vi "Resolution effect on SFDR.vi"() -> ()   [LabVIEW 2019]
uses:
  <vilib>/Analysis/4window.llb/windowTd.ctl
  <vilib>/measure/maspectr.llb/Power Spectrum and PSD Export Mode.ctl
  <vilib>/measure/maspectr.llb/FFT Power Spectrum and PSD for N Chan.vi
  <vilib>/measure/NI_MABase.lvlib
  <vilib>/measure/NI_MAPro.lvlib
  <vilib>/Analysis/NI_AALPro.lvlib
panel:
  out "Power spectrum":cluster{"f0":dbl, "df":dbl, "magnitude":dbl[]}[](graph)
  in  "sampling info":cluster{"Fs":dbl, "#s":dbl}={"Fs"=3072000000.0, "#s"=16000.0}
  in  "amplitude":dbl=0.5 format="%0.2p"
  in  "Fc":dbl=500000000.0 format="%#_6pHz"
  out "noise level":dbl=-81.98970004336019 format="%#_gdbm"
  in  "BW":dbl=2000000000.0 format="%#_6pHz"
  in  "Noise density":dbl=-155.0 format="%#_gdbm/Hz"
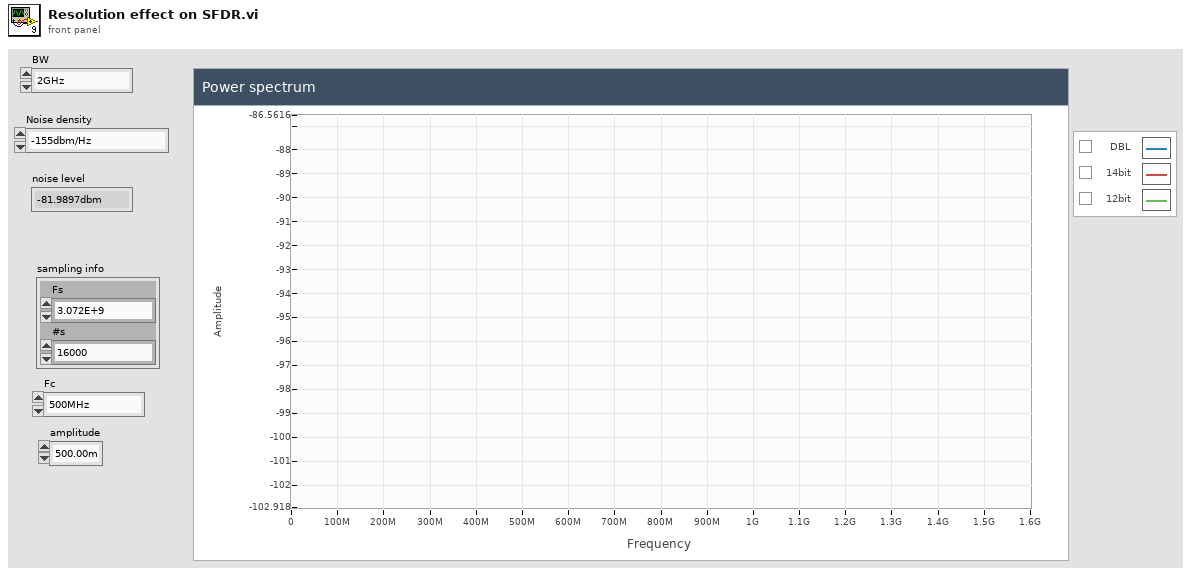
[diagram p1: front panel]
types:
  T1 = typedef "NI_MAPro.lvlib/Power Spectrum and PSD Export Mode.ctl" = u16
  T2 = typedef "NI_AALPro.lvlib/windowTd.ctl" = u32
  T3 = enum16{"Sine Wave", "Triangle Wave", "Square Wave", "Sawtooth Wave"}
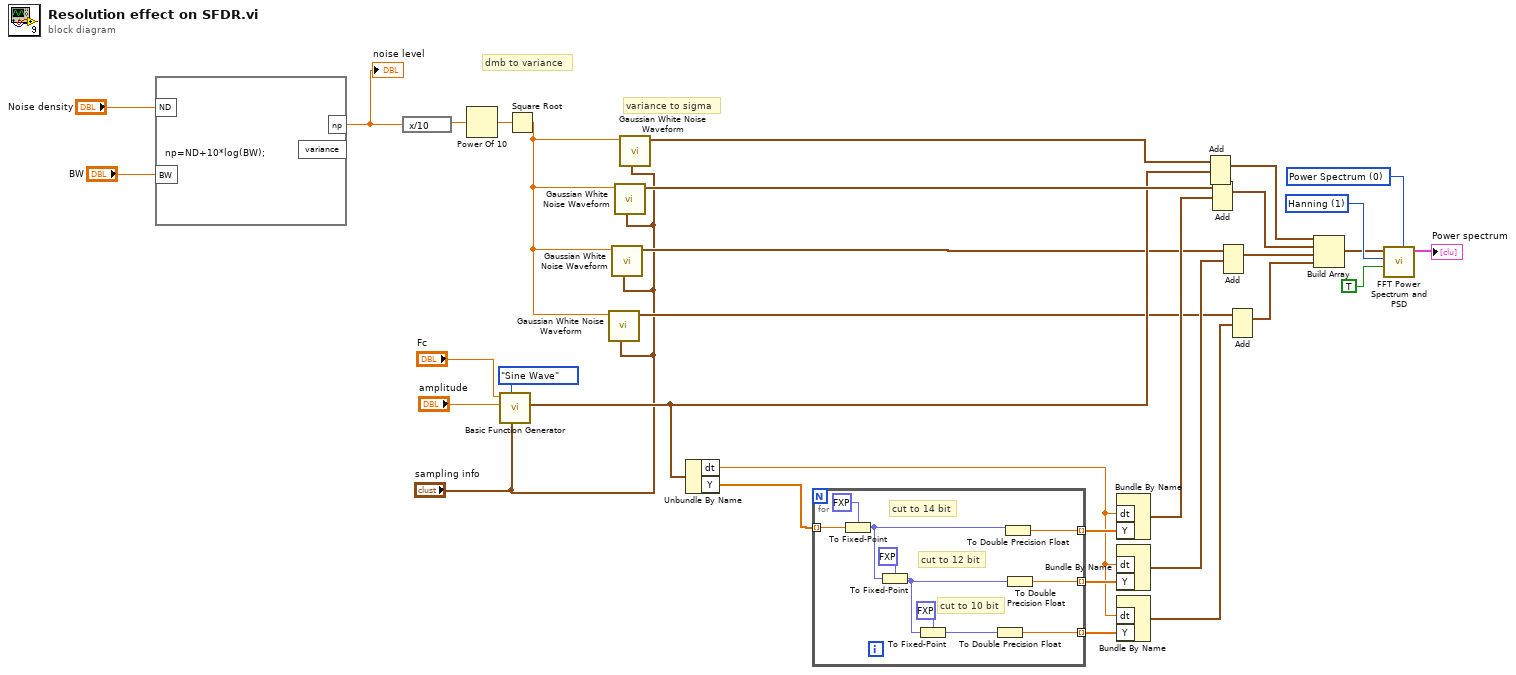
[diagram p0: block diagram]
diagram:
  w22 = T1 0 items=["Power Spectrum", "Power Spectral Density"] ("export mode")
  w24 = T2 1 items=["Rectangle"=0, "Hanning"=1, "Hamming"=2, "Blackman-Harris"=3, "Exact Blackman"=4, "Blackman"=5, "Flat Top"=6, "4 Term B-Harris "=7, "7 Term B-Harris"=8, "Low Sidelobe"=9, "Blackman Nuttall"=11, "Triangle"=30, "Bartlett-Hanning"=31, "Bohman"=32, "Parzen"=33, "Welch"=34, "Kaiser"=60, "Dolph-Chebyshev"=61, "Gaussian"=62] ("window")
  # "variance to sigma"
  # "dmb to variance"
  n1 = formula code="np=ND+10*log(BW);"("ND"="Noise density", "BW"="BW") -> ("np"=w30:dbl)  [unwired: 1 out]
  "noise level" <- w30
  n2 = expression code="x/10"(w30) -> (w29:dbl)
  n3 = Power Of 10(x=w29) -> (10^x=w28:dbl)
  n4 = call <vilib>:"Basic Function Generator.vi"("sampling info"="sampling info", "signal type"=T3."Sine Wave", "amplitude"="amplitude", "frequency"="Fc") -> ("signal out"=w14:waveform(dbl))  [unwired: 5 in, 2 out]
  n5 = Square Root(x=w28) -> (sqrt(x)=w8:dbl)
  n6 = call <vilib>:"Gaussian White Noise Waveform.vi"("sampling info"="sampling info", "standard deviation"=w8) -> ("signal out"=w5:waveform(dbl))  [unwired: 8 in, 1 out]
  n7 = call <vilib>:"Gaussian White Noise Waveform.vi"("sampling info"="sampling info", "standard deviation"=w8) -> ("signal out"=w12:waveform(dbl))  [unwired: 8 in, 1 out]
  n8 = call <vilib>:"Gaussian White Noise Waveform.vi"("sampling info"="sampling info", "standard deviation"=w8) -> ("signal out"=w16:waveform(dbl))  [unwired: 8 in, 1 out]
  n9 = call <vilib>:"Gaussian White Noise Waveform.vi"("sampling info"="sampling info", "standard deviation"=w8) -> ("signal out"=w19:waveform(dbl))  [unwired: 8 in, 1 out]
  n10 = Unbundle By Name(w14) -> ("dt"=w2:dbl, "Y"=w15:dbl[])
  n11 = for {
    tunnel: w15 -> [w42] mode=indexing
    tunnel: [w40] -> w18 mode=indexing
    tunnel: [w37] -> w13 mode=indexing
    tunnel: [w33] -> w6 mode=indexing
    # "cut to 10 bit"
    # "cut to 12 bit"
    # "cut to 14 bit"
    n12 = To Fixed-Point(fixed-point type=fxp<+/-,14,1> 0.0, number=w42) -> (fixed-point=w38:fxp<+/-,14,1>)
    n13 = To Fixed-Point(fixed-point type=fxp<+/-,12,1> 0.0, number=w38) -> (fixed-point=w35:fxp<+/-,12,1>)
    n14 = To Fixed-Point(fixed-point type=fxp<+/-,10,1> 0.0, number=w35) -> (fixed-point=w34:fxp<+/-,10,1>)
    n15 = To Double Precision Float(number=w34) -> (double precision float=w33:dbl)
    n16 = To Double Precision Float(number=w38) -> (double precision float=w40:dbl)
    n17 = To Double Precision Float(number=w35) -> (double precision float=w37:dbl)
  }
  n18 = Bundle By Name("dt"=w2, "Y"=w18) -> (w17:waveform(dbl))  [unwired: 1 in]
  n19 = Bundle By Name("dt"=w2, "Y"=w13) -> (w7:waveform(dbl))  [unwired: 1 in]
  n20 = Bundle By Name("dt"=w2, "Y"=w6) -> (w4:waveform(dbl))  [unwired: 1 in]
  n21 = Add(1:w14, 2:w19) -> (0:w20:waveform(dbl))  [unwired: 1 in, 1 out]
  n22 = Add(1:w17, 2:w16) -> (0:w10:waveform(dbl))  [unwired: 1 in, 1 out]
  n23 = Add(1:w7, 2:w12) -> (0:w9:waveform(dbl))  [unwired: 1 in, 1 out]
  n24 = Add(1:w4, 2:w5) -> (0:w3:waveform(dbl))  [unwired: 1 in, 1 out]
  n25 = Build Array(w20, w10, w9, w3) -> (w11:waveform(dbl)[])
  n26 = call-poly <vilib>:"FFT Power Spectrum and PSD.vi"("export mode"=w22, "dB On (F)"=TRUE, "window"=w24, "time signals"=w11) -> ("Power Spectrum / PSD"=→"Power spectrum":cluster{"f0":dbl, "df":dbl, "magnitude":dbl[]}[])  [unwired: 4 in, 3 out]
